vi "UIRef.vi"(8 "error in":errorcluster, 11 "bin datalogger editor node in":refnum<class "Binary datalogger editor node.lvclass">) -> (0 "error out":errorcluster, 2 "VI refnum":refnum<vi>, 3 "bin datalogger editor node out":refnum<class "Binary datalogger editor node.lvclass">)   [LabVIEW 2013, in "Binary datalogger editor node.lvclass"]
uses:
  Binary datalogger editor node.lvclass
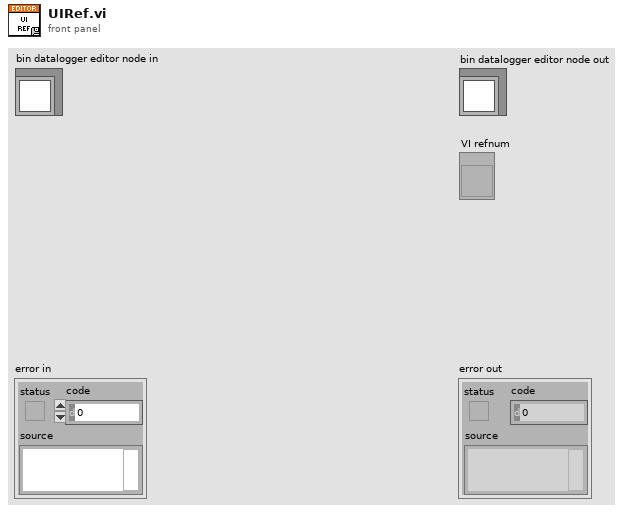
[diagram p1: front panel]
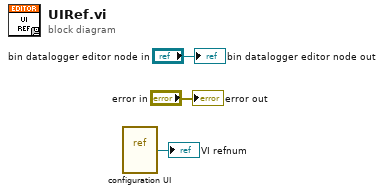
[diagram p0: block diagram]
diagram:
  n1 = vi-ref "configuration UI.vi"() -> (→"VI refnum":refnum<vi>)
  "error out" <- "error in"
  "bin datalogger editor node out" <- "bin datalogger editor node in"
